vi "Get Data.vi"(8 "error in (no error)":errorcluster, 11 "TECData in":refnum<class "TECData.lvclass">) -> (0 "error out":errorcluster, 1 "Power":sgl, 2 "T":sgl, 3 "TECData out":refnum<class "TECData.lvclass">)   [LabVIEW 2015, in "TE Cooler.lvlib" / "TECData.lvclass"]
doc: "Retrieve the data for the thermoelectric cooler. The T is the temperature and power is the amount of power that the TEC is using to cool or heat the device."
uses:
  TECData.lvclass
  TECData.lvclass/TECData.ctl
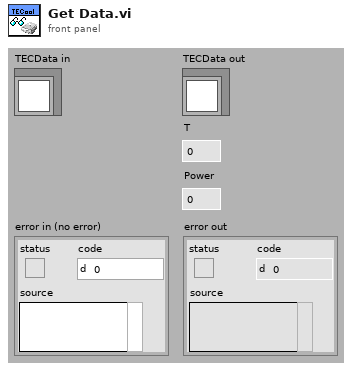
[diagram p1: front panel]
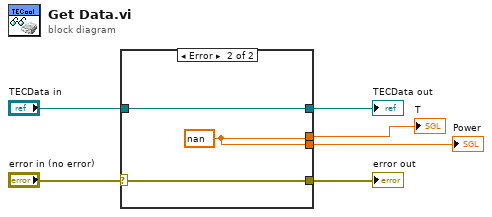
[diagram p0: block diagram]
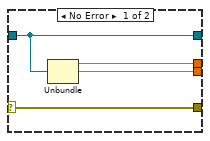
[diagram p2: hidden frame]
diagram:
  n1 = case shown="Error" "error in (no error)" {
    selector: "error in (no error)" -> [w10 w13]
    tunnel: [w10 w13] -> w5
    tunnel: [w9 w12] -> w3
    tunnel: "TECData in" -> [w9 w12]
    tunnel: [w8 w11] -> w2
    tunnel: [w7 w11] -> w1
    frame No Error {
      n2 = Unbundle(w9) -> (w8:sgl, w7:sgl)  [unwired: 1 out]
    }
    frame Error {
      w11 = nan ("T")
    }
  }
  "error out" <- w5
  "TECData out" <- w3
  "T" <- w2
  "Power" <- w1
